vi "TEST - Object Recursion.vi"(8 "error in (no error)":errorcluster) -> (0 "error out":errorcluster, 2 "pass":bool)   [LabVIEW 2020, in "test_openg_array.lvlib"]
uses:
  test_openg_array.lvlib
  LVOOP Data/Top Level Class/Top Level Data.lvclass
  LVOOP Data/Subclass Data/Subclass Data.lvclass
  source/library/openg_variant.lvlib
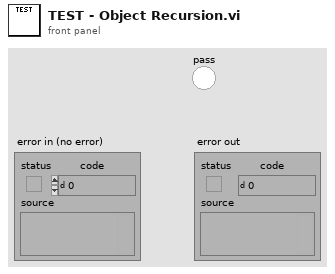
[diagram p1: front panel]
types:
  T1 = cluster{"Numeric":i32, "String":string, "Subclass Data":refnum<class "Subclass Data.lvclass">}
  T2 = cluster{"Numeric":i32, "String":string, "Subcluster":cluster{"Boolean":bool, "Path":path}}
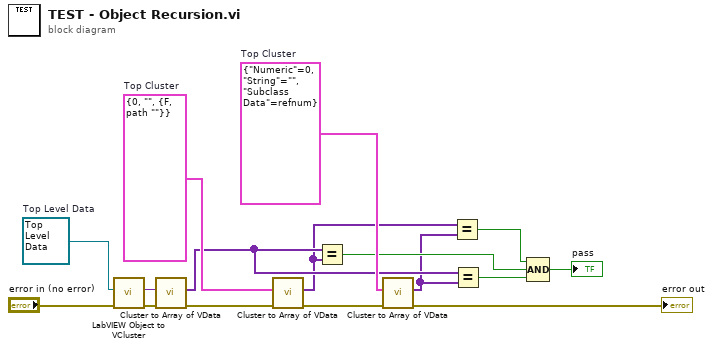
[diagram p0: block diagram]
diagram:
  w9 = T1 {"Numeric"=0, "String"="", "Subclass Data"=refnum}  # Top Cluster
  w14 = T2 {"Numeric"=0, "String"="", "Subcluster"={"Boolean"=FALSE, "Path"=path ""}}  # Top Cluster
  w16 = refnum<class "Top Level Data.lvclass"> refnum  # Top Level Data
  n1 = call "LabVIEW Object to VCluster.vi"("error in (no error)"="error in (no error)", "LabVIEW Object"=w16) -> ("error out"=w13:errorcluster, "VCluster"=w15:variant)  [unwired: 8 in]
  n2 = call "Cluster to Array of VData.vi"("error in (no error)"=w13, "Cluster"=w15) -> ("error out"=w11:errorcluster, "Array of VData"=w8:variant[])  [unwired: 8 in]
  n3 = call "Cluster to Array of VData.vi"("error in (no error)"=w11, "Cluster"=w14) -> ("error out"=w10:errorcluster, "Array of VData"=w2:variant[])  [unwired: 8 in]
  n4 = Equal?(x=w8, y=w2) -> (x = y?=w5:bool)
  n5 = call "Cluster to Array of VData.vi"("error in (no error)"=w10, "Cluster"=w9) -> ("error out"=→"error out":errorcluster, "Array of VData"=w3:variant[])  [unwired: 8 in]
  n6 = Equal?(x=w2, y=w3) -> (x = y?=w1:bool)
  n7 = Equal?(x=w8, y=w3) -> (x = y?=w6:bool)
  n8 = Compound Arithmetic op=AND(w1, w5, w6) -> (→"pass":bool)
